vi "Decrypt.vi"(11 "String":string) -> (3 "Output String":string)   [LabVIEW 2013]
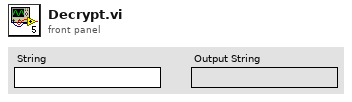
[diagram p1: front panel]
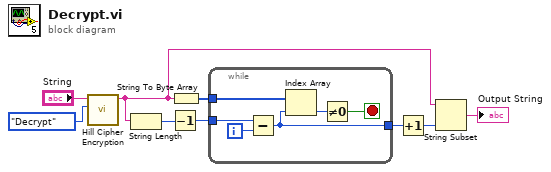
[diagram p0: block diagram]
diagram:
  n1 = call <userlib>:"Hill Cipher Encryption.vi"("Operation"=enum16{"Encrypt", "Decrypt", "Decrypt from Hex"}."Decrypt", "Input String"="String") -> ("Output String"=w8:string)  [unwired: 7 in, 2 out]
  n2 = String Length(string=w8) -> (length=w4:i32)
  n3 = Decrement(x=w4) -> (x-1=w5:i32)
  n4 = String To Byte Array(string=w8) -> (unsigned byte array=w3:u8[])
  n5 = while {
    tunnel: w3 -> [w13]
    tunnel: w5 -> [w14]
    tunnel: [w10] -> w6
    i -> [w15]
    stop <- w12 stop-if-true
    n6 = Subtract(x=w14, y=w15) -> (x-y=w10:i32)
    n7 = Index Array(array=w13, index=w10) -> (element=w11:u8)
    n8 = Not Equal To 0?(x=w11) -> (x != 0?=w12:bool)
  }
  n9 = Increment(x=w6) -> (x+1=w7:i32)
  n10 = String Subset(string=w8, length (rest)=w7) -> (substring=→"Output String":string)  [unwired: 1 in]
